vi "HeatFlow Conf HW.vi"(9 "HeatFlowHW Cfg":T1) -> (0 "error out":errorcluster, 3 "Hardware Tasks out":T2)   [LabVIEW 2019, in "Acquisition.lvlib"]
doc: "Initialize the hardware references."
uses:
  Acquisition.lvlib
  HeatFlow HW Tasks.ctl
  HeatFlow HW Cfg.ctl
  HeatFlow Acq States.ctl
  <vilib>/DAQmx/create/channels.llb/DAQmx Create Channel (AI-Voltage-Basic).vi
  <vilib>/Instr/_visa.llb/VISA Configure Serial Port (Instr).vi
  <vilib>/DAQmx/create/channels.llb/DAQmx Create Channel (AI-Temperature-RTD).vi
  <vilib>/DAQmx/create/channels.llb/DAQmx Create Channel (AO-Voltage-Basic).vi
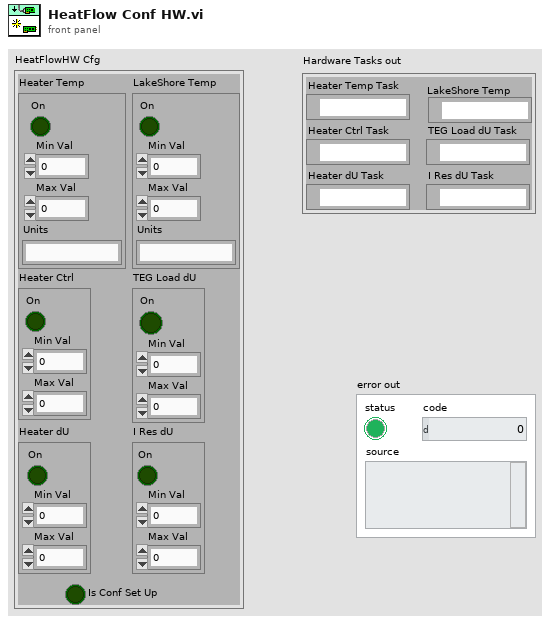
[diagram p1: front panel]
types:
  T1 = typedef "Acquisition.lvlib/HeatFlow HW Cfg.ctl" = cluster{"Heater Temp":cluster{"On":bool, "Min Val":dbl, "Max Val":dbl, "Units":string}, "LakeShore Temp":cluster{"On":bool, "Min Val":dbl, "Max Val":dbl, "Units":string}, "Heater Ctrl":cluster{"On":bool, "Min Val":dbl, "Max Val":dbl}, "TEG Load dU":cluster{"On":bool, "Min Val":dbl, "Max Val":dbl}, "Heater dU":cluster{"On":bool, "Min Val":dbl, "Max Val":dbl}, "I Res dU":cluster{"On":bool, "Min Val":dbl, "Max Val":dbl}, "Is Conf Set Up":bool}
  T2 = typedef "Acquisition.lvlib/HeatFlow HW Tasks.ctl" = cluster{"Heater Temp Task":refnum<k21>, "Heater Ctrl Task":refnum<k21>, "TEG Load dU Task":refnum<k21>, "Heater dU Task":refnum<k21>, "I Res dU Task":refnum<k21>, "LakeShore Temp":refnum<visa-resource-name>}
  T3 = typedef "Acquisition.lvlib/HeatFlow Acq States.ctl" = enum16{"Start", "--- Control ---", "HeaterTemp", "DoControl?", "HeaterCtrl", "--- Readings ---", "DoReadings?", "I_Res_dU", "LakeShoreTemp", "Heater_dU", "TEG_Load_dU", "Calculations", "End"}
  T4 = cluster{"On":bool, "Min Val":dbl, "Max Val":dbl, "Units":string}
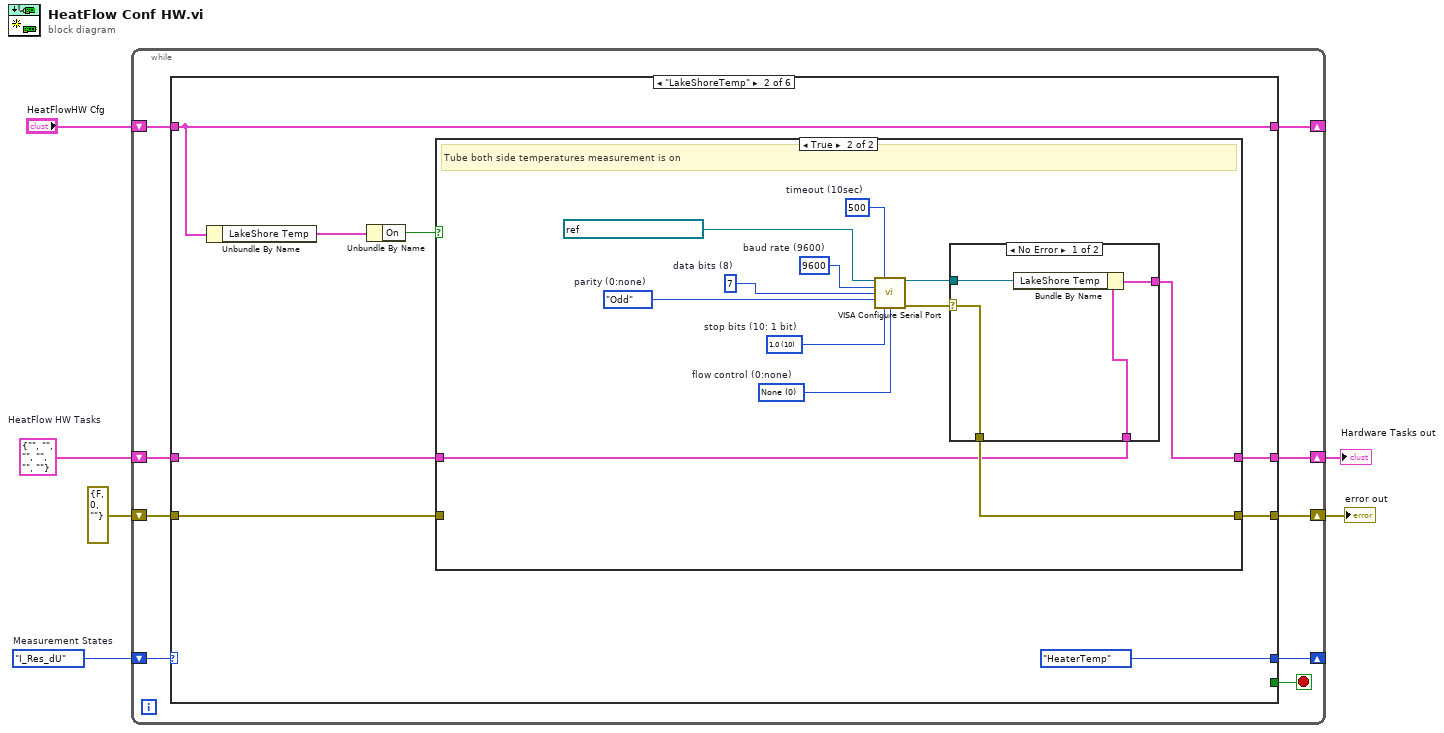
[diagram p0: block diagram]
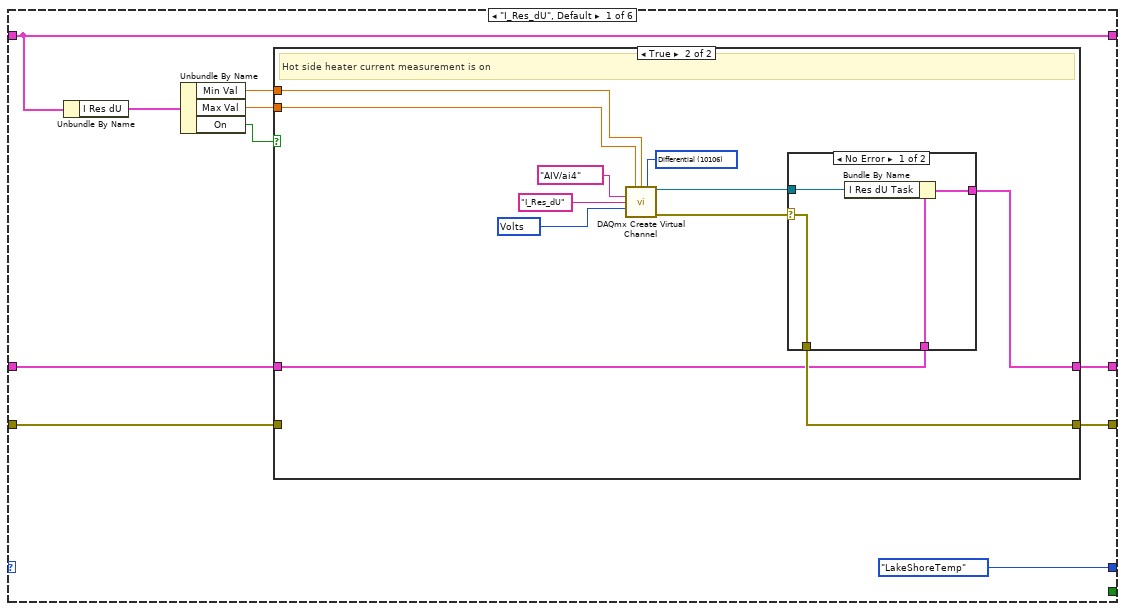
[diagram p2: hidden frame]
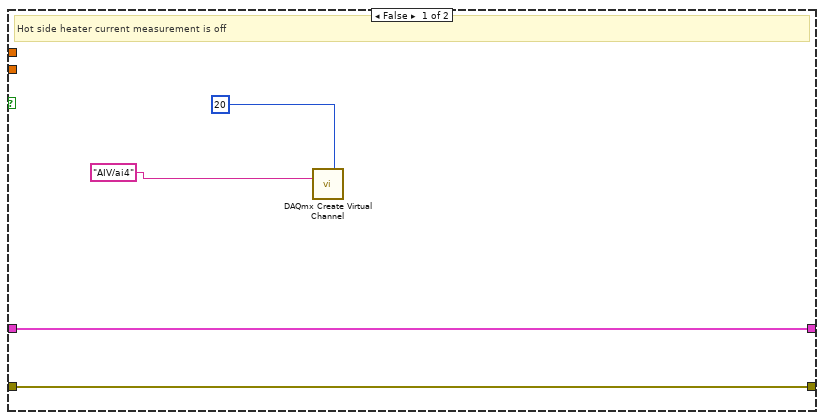
[diagram p3: hidden frame]
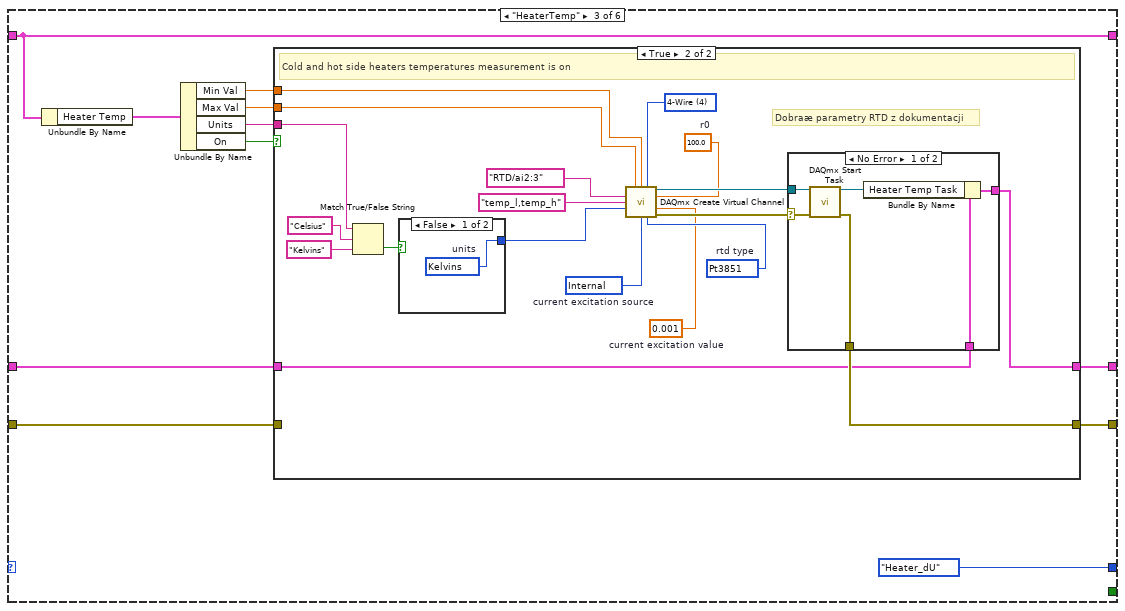
[diagram p7: hidden frame]
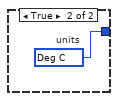
[diagram p9: hidden frame]
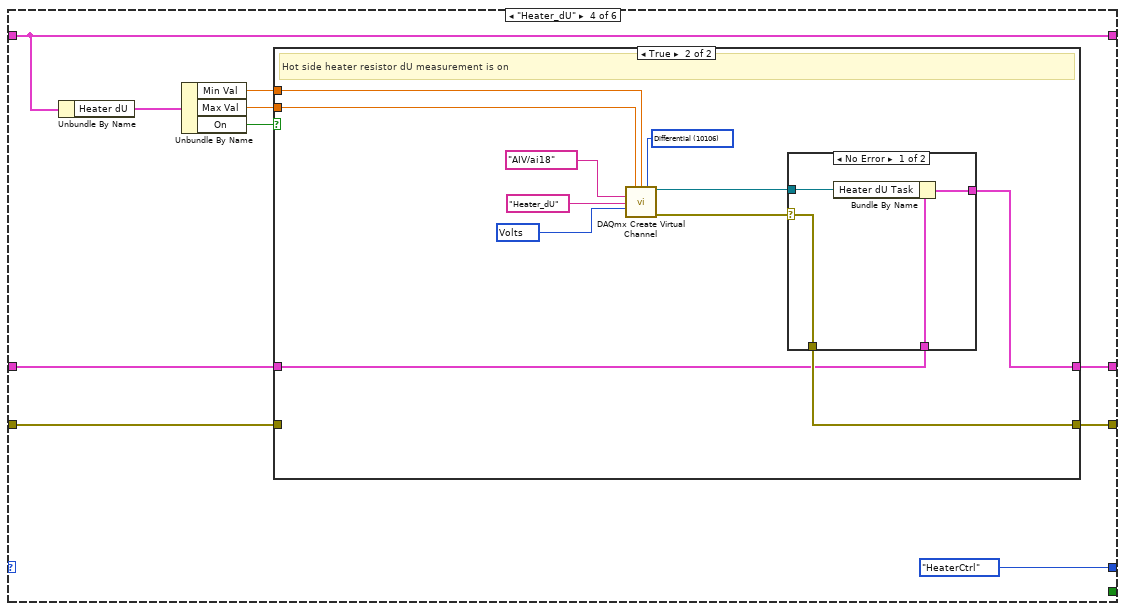
[diagram p11: hidden frame]
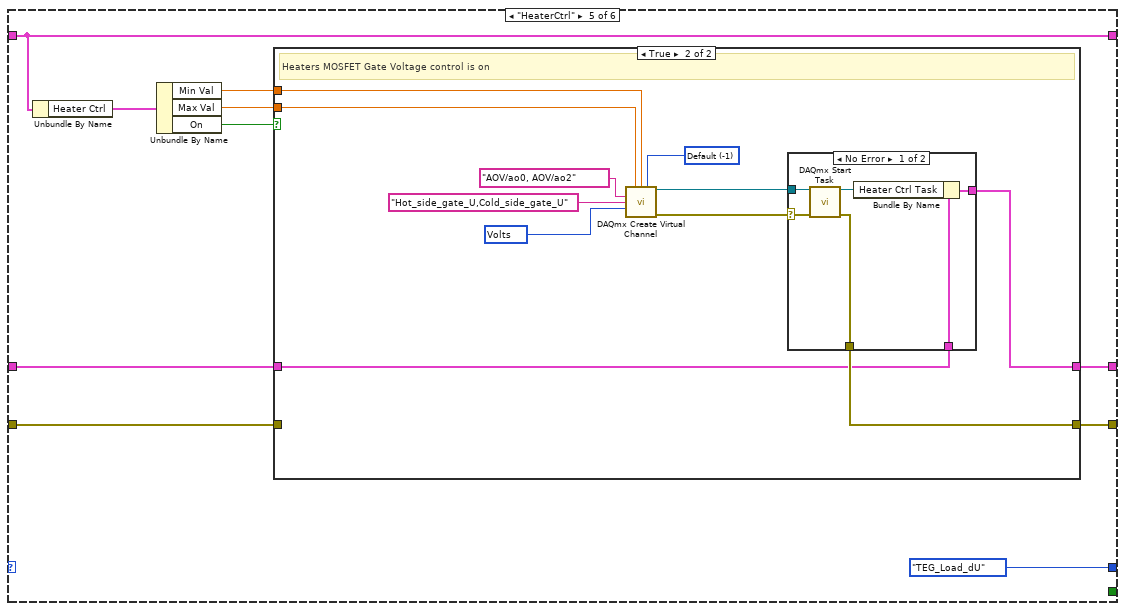
[diagram p14: hidden frame]
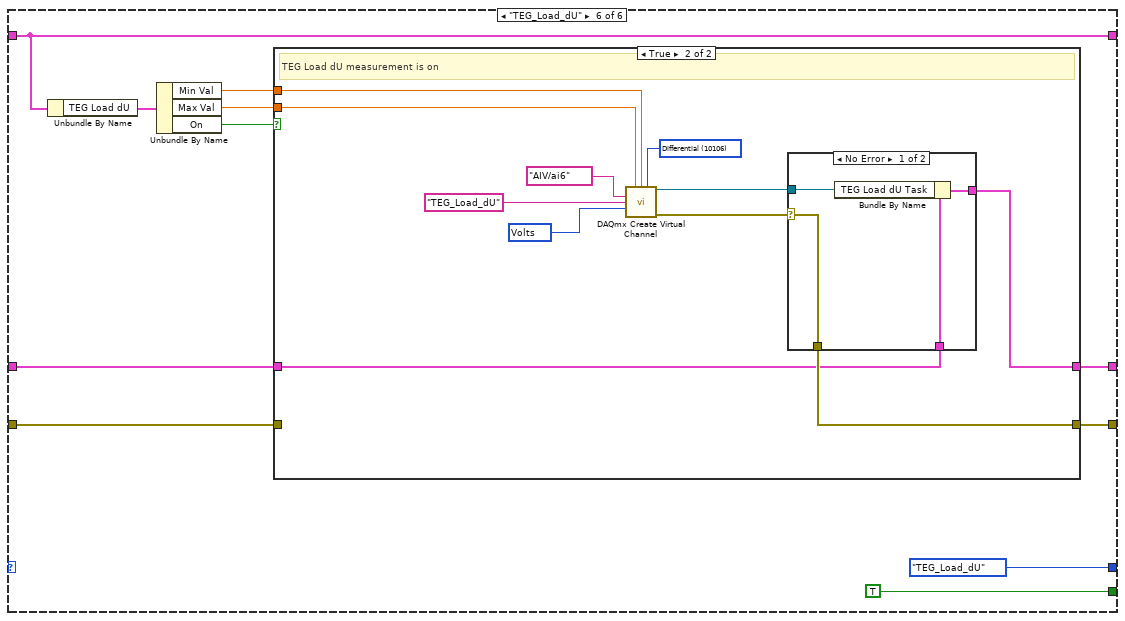
[diagram p17: hidden frame]
diagram:
  w5 = T2 {"Heater Temp Task"="", "Heater Ctrl Task"="", "TEG Load dU Task"="", "Heater dU Task"="", "I Res dU Task"="", "LakeShore Temp"=""}  # HeatFlow HW Tasks
  w6 = HeatFlow_Acq_States."I_Res_dU"  # Measurement States
  n1 = while {
    shift-right: [w14] -> _
    shift-left: w6 -> [w15]
    shift-right: [w12] -> _
    shift-left: "HeatFlowHW Cfg" -> [w13]
    shift-right: [w7] -> w2
    shift-left: w5 -> [w10]
    shift-right: [w8] -> w3
    shift-left: errorcluster {"status"=FALSE, "code"=0, "source"=""} ("error out") -> [w9]
    stop <- w11 stop-if-true
    n2 = case shown="\"LakeShoreTemp\"" w15 {
      tunnel: [HeatFlow_Acq_States."LakeShoreTemp" ("Measurement States") HeatFlow_Acq_States."HeaterTemp" ("Measurement States") HeatFlow_Acq_States."Heater_dU" ("Measurement States") HeatFlow_Acq_States."HeaterCtrl" ("Measurement States") HeatFlow_Acq_States."TEG_Load_dU" ("Measurement States") HeatFlow_Acq_States."TEG_Load_dU" ("Measurement States")] -> w14
      tunnel: w13 -> [w18 w48 w76 w125 w154 w186]
      tunnel: [w18 w48 w76 w125 w154 w186] -> w12
      tunnel: [_ _ _ _ _ TRUE] -> w11
      tunnel: w10 -> [w24 w52 w83 w124 w153 w185]
      tunnel: w9 -> [w21 w51 w79 w121 w150 w182]
      tunnel: [w20 w50 w78 w120 w149 w181] -> w8
      tunnel: [w19 w49 w77 w119 w148 w180] -> w7
      frame "I_Res_dU", Default {
        n3 = Unbundle By Name(w18) -> ("I Res dU"=w17:cluster{"On":bool, "Min Val":dbl, "Max Val":dbl})
        n4 = Unbundle By Name(w17) -> ("Min Val"=w23:dbl, "Max Val"=w22:dbl, "On"=w16:bool)
        n5 = case shown="True" w16 {
          tunnel: w24 -> [w29 w33]
          tunnel: w23 -> [_ w37]
          tunnel: w22 -> [_ w36]
          tunnel: w21 -> [w28 _]
          tunnel: [w28 w35] -> w20
          tunnel: [w29 w34] -> w19
          frame False {
            # "Hot side heater current measurement is off"
            n6 = call-poly <vilib>:"DAQmx Create Virtual Channel.vi"("input terminal configuration"=20, "physical channels"="AIV/ai4") -> ()  [unwired: 12 in, 2 out]
          }
          frame True {
            w30 = 10106 items=["Default"=-1, "RSE"=10083, "NRSE"=10078, "Differential"=10106, "Pseudodifferential"=12529] ("input terminal configuration")
            w31 = 10348 items=["Volts"=10348, "From Custom Scale"=10065] ("units")
            # "Hot side heater current measurement is on"
            n7 = call-poly <vilib>:"DAQmx Create Virtual Channel.vi"("maximum value"=w36, "minimum value"=w37, "input terminal configuration"=w30, "physical channels"=tag "AIV/ai4", "name to assign"="I_Res_dU", "units"=w31) -> ("task out"=w39:refnum<k21>, "error out"=w40:errorcluster)  [unwired: 8 in]
            n8 = case shown="No Error" w40 {
              selector: w40 -> [w41 w46]
              tunnel: w39 -> [w42 _]
              tunnel: [w41 w46] -> w35
              tunnel: [w44 w45] -> w34
              tunnel: w33 -> [w43 w45]
              frame No Error {
                n9 = Bundle By Name(cluster=w43, "I Res dU Task"=w42) -> (w44:T2)
              }
              frame Error {
              }
            }
          }
        }
      }
      frame "LakeShoreTemp" {
        n10 = Unbundle By Name(w48) -> ("LakeShore Temp"=w47:T4)
        n11 = Unbundle By Name(w47) -> ("On"=w53:bool)
        n12 = case shown="True" w53 {
          tunnel: w52 -> [w56 w66]
          tunnel: w51 -> [w55 _]
          tunnel: [w55 w68] -> w50
          tunnel: [w56 w67] -> w49
          frame False {
            # "Tube both side temperatures measurement is off"
          }
          frame True {
            w57 = u32 500  # timeout (10sec)
            w58 = u16 0 items=["None", "XON/XOFF", "RTS/CTS", "XON/XOFF & RTS/CTS", "DTR/DSR", "XON/XOFF & DTR/DSR"]  # flow control (0:none)
            w59 = u16 10 items=["1.0"=10, "1.5"=15, "2.0"=20]  # stop bits (10: 1 bit)
            w60 = enum16{"None", "Odd", "Even", "Mark", "Space"}."Odd"  # parity (0:none)
            w61 = u16 7  # data bits (8)
            w62 = u32 9600  # baud rate (9600)
            # "Tube both side temperatures measurement is on"
            n13 = call-poly "VISA Configure Serial Port"("VISA resource name"=refnum<visa-resource-name> "COM2_TempMonitor", "timeout (10sec)"=w57, "baud rate (9600)"=w62, "data bits (8)"=w61, "parity (0:none)"=w60, "stop bits (10: 1 bit)"=w59, "flow control (0:none)"=w58) -> ("VISA resource name out"=w64:refnum<visa-resource-name>, "error out"=w65:errorcluster)  [unwired: 7 in]
            n14 = case shown="No Error" w65 {
              selector: w65 -> [w70 w74]
              tunnel: [w70 w74] -> w68
              tunnel: [w72 w73] -> w67
              tunnel: w66 -> [w71 w73]
              tunnel: w64 -> [w69 _]
              frame No Error {
                n15 = Bundle By Name(cluster=w71, "LakeShore Temp"=w69) -> (w72:T2)
              }
              frame Error {
              }
            }
          }
        }
      }
      frame "HeaterTemp" {
        n16 = Unbundle By Name(w76) -> ("Heater Temp"=w75:T4)
        n17 = Unbundle By Name(w75) -> ("Min Val"=w82:dbl, "Max Val"=w81:dbl, "Units"=w80:string, "On"=w84:bool)
        n18 = case shown="True" w84 {
          tunnel: w83 -> [w87 w89]
          tunnel: w82 -> [_ w98]
          tunnel: w81 -> [_ w97]
          tunnel: w80 -> [_ w93]
          tunnel: w79 -> [w86 _]
          tunnel: [w86 w91] -> w78
          tunnel: [w87 w90] -> w77
          frame False {
            # "Cold and hot side heaters temperatures measurement is off"
          }
          frame True {
            w88 = 0.001  # current excitation value
            w100 = 10200 items=["Internal"=10200, "External"=10167, "None"=10230]  # current excitation source
            w102 = 100.0  # r0
            w104 = 4 items=["2-Wire"=2, "3-Wire"=3, "4-Wire"=4] ("resistance configuration")
            w99 = 10071 items=["Pt3750"=12481, "Pt3851"=10071, "Pt3911"=12482, "Pt3916"=10069, "Pt3920"=10053, "Pt3928"=12483, "Custom"=10137]  # rtd type
            # "Dobraæ parametry RTD z dokumentacji"
            # "Cold and hot side heaters temperatures measurement is on"
            n19 = Match True/False String(2:"Kelvins" ("false string"), 3:"Celsius" ("true string"), 4:w93) -> (0:w94:bool)  [unwired: 1 out]
            n20 = case shown="False" w94 {
              tunnel: [w107 w108] -> w92
              frame False {
                w107 = 10325 items=["Deg C"=10143, "Deg F"=10144, "Kelvins"=10325, "Deg R"=10145, "From Custom Scale"=10065]  # units
              }
              frame True {
                w108 = 10143 items=["Deg C"=10143, "Deg F"=10144, "Kelvins"=10325, "Deg R"=10145, "From Custom Scale"=10065]  # units
              }
            }
            n21 = call-poly <vilib>:"DAQmx Create Virtual Channel.vi"("maximum value"=w97, "minimum value"=w98, "resistance configuration"=w104, "physical channels"=tag "RTD/ai2:3", "r0"=w102, "name to assign"="temp_l,temp_h", "units"=w92, "current excitation value"=w88, "current excitation source"=w100, "rtd type"=w99) -> ("task out"=w105:refnum<k21>, "error out"=w106:errorcluster)  [unwired: 4 in]
            n22 = case shown="No Error" w106 {
              selector: w106 -> [w112 w116]
              tunnel: w105 -> [w114 _]
              tunnel: [w111 w116] -> w91
              tunnel: [w110 w115] -> w90
              tunnel: w89 -> [w109 w115]
              frame No Error {
                n23 = call <vilib>:"DAQmx Start Task.vi"("task/channels in"=w114, "error in"=w112) -> ("task out"=w113:refnum<k21>, "error out"=w111:errorcluster)  [unwired: 12 in]
                n24 = Bundle By Name(cluster=w109, "Heater Temp Task"=w113) -> (w110:T2)
              }
              frame Error {
              }
            }
          }
        }
      }
      frame "Heater_dU" {
        n25 = Unbundle By Name(w125) -> ("Heater dU"=w118:cluster{"On":bool, "Min Val":dbl, "Max Val":dbl})
        n26 = Unbundle By Name(w118) -> ("Min Val"=w123:dbl, "Max Val"=w122:dbl, "On"=w117:bool)
        n27 = case shown="True" w117 {
          tunnel: w124 -> [w128 w131]
          tunnel: w123 -> [_ w135]
          tunnel: w122 -> [_ w134]
          tunnel: w121 -> [w127 _]
          tunnel: [w127 w133] -> w120
          tunnel: [w128 w132] -> w119
          frame False {
            # "Hot side heater resistor dU measurement is off"
          }
          frame True {
            w129 = 10106 items=["Default"=-1, "RSE"=10083, "NRSE"=10078, "Differential"=10106, "Pseudodifferential"=12529] ("input terminal configuration")
            w130 = 10348 items=["Volts"=10348, "From Custom Scale"=10065] ("units")
            # "Hot side heater resistor dU measurement is on"
            n28 = call-poly <vilib>:"DAQmx Create Virtual Channel.vi"("maximum value"=w134, "minimum value"=w135, "input terminal configuration"=w129, "physical channels"=tag "AIV/ai18", "name to assign"="Heater_dU", "units"=w130) -> ("task out"=w138:refnum<k21>, "error out"=w139:errorcluster)  [unwired: 8 in]
            n29 = case shown="No Error" w139 {
              selector: w139 -> [w140 w145]
              tunnel: w138 -> [w141 _]
              tunnel: [w140 w145] -> w133
              tunnel: [w143 w144] -> w132
              tunnel: w131 -> [w142 w144]
              frame No Error {
                n30 = Bundle By Name(cluster=w142, "Heater dU Task"=w141) -> (w143:T2)
              }
              frame Error {
              }
            }
          }
        }
      }
      frame "HeaterCtrl" {
        n31 = Unbundle By Name(w154) -> ("Heater Ctrl"=w147:cluster{"On":bool, "Min Val":dbl, "Max Val":dbl})
        n32 = Unbundle By Name(w147) -> ("Min Val"=w152:dbl, "Max Val"=w151:dbl, "On"=w146:bool)
        n33 = case shown="True" w146 {
          tunnel: w153 -> [w157 w161]
          tunnel: w152 -> [_ w165]
          tunnel: w151 -> [_ w164]
          tunnel: w150 -> [w156 _]
          tunnel: [w156 w163] -> w149
          tunnel: [w157 w162] -> w148
          frame False {
            # "Heaters MOSFET Gate Voltage control is off"
          }
          frame True {
            w158 = -1 items=["Default"=-1, "RSE"=10083, "Differential"=10106, "Pseudodifferential"=12529] ("output terminal configuration")
            w159 = 10348 items=["Volts"=10348, "From Custom Scale"=10065] ("units")
            # "Heaters MOSFET Gate Voltage control is on"
            n34 = call-poly <vilib>:"DAQmx Create Virtual Channel.vi"("maximum value"=w164, "minimum value"=w165, "output terminal configuration"=w158, "physical channels"=tag "AOV/ao0, AOV/ao2", "name to assign"="Hot_side_gate_U,Cold_side_gate_U", "units"=w159) -> ("task out"=w167:refnum<k21>, "error out"=w168:errorcluster)  [unwired: 8 in]
            n35 = case shown="No Error" w168 {
              selector: w168 -> [w172 w176]
              tunnel: w167 -> [w174 _]
              tunnel: [w171 w176] -> w163
              tunnel: [w170 w175] -> w162
              tunnel: w161 -> [w169 w175]
              frame No Error {
                n36 = call <vilib>:"DAQmx Start Task.vi"("task/channels in"=w174, "error in"=w172) -> ("task out"=w173:refnum<k21>, "error out"=w171:errorcluster)  [unwired: 12 in]
                n37 = Bundle By Name(cluster=w169, "Heater Ctrl Task"=w173) -> (w170:T2)
              }
              frame Error {
              }
            }
          }
        }
      }
      frame "TEG_Load_dU" {
        n38 = Unbundle By Name(w186) -> ("TEG Load dU"=w178:cluster{"On":bool, "Min Val":dbl, "Max Val":dbl})
        n39 = Unbundle By Name(w178) -> ("Min Val"=w184:dbl, "Max Val"=w183:dbl, "On"=w177:bool)
        n40 = case shown="True" w177 {
          tunnel: w185 -> [w189 w194]
          tunnel: w184 -> [_ w198]
          tunnel: w183 -> [_ w197]
          tunnel: w182 -> [w188 _]
          tunnel: [w188 w196] -> w181
          tunnel: [w189 w195] -> w180
          frame False {
            # "TEG Load dU measurement is off"
          }
          frame True {
            w190 = 10106 items=["Default"=-1, "RSE"=10083, "NRSE"=10078, "Differential"=10106, "Pseudodifferential"=12529] ("input terminal configuration")
            w191 = 10348 items=["Volts"=10348, "From Custom Scale"=10065] ("units")
            # "TEG Load dU measurement is on"
            n41 = call-poly <vilib>:"DAQmx Create Virtual Channel.vi"("maximum value"=w197, "minimum value"=w198, "input terminal configuration"=w190, "physical channels"=tag "AIV/ai6", "name to assign"="TEG_Load_dU", "units"=w191) -> ("task out"=w199:refnum<k21>, "error out"=w200:errorcluster)  [unwired: 8 in]
            n42 = case shown="No Error" w200 {
              selector: w200 -> [w201 w206]
              tunnel: w199 -> [w202 _]
              tunnel: [w201 w206] -> w196
              tunnel: [w204 w205] -> w195
              tunnel: w194 -> [w203 w205]
              frame No Error {
                n43 = Bundle By Name(cluster=w203, "TEG Load dU Task"=w202) -> (w204:T2)
              }
              frame Error {
              }
            }
          }
        }
      }
    }
  }
  "error out" <- w3
  "Hardware Tasks out" <- w2
